vi "Launcher.vi"(8 "error in (no error)":errorcluster) -> (0 "error out":errorcluster)   [LabVIEW 2022 SP3]
doc: "This VI launches the image analyzer application."
uses:
  Controls/LauncherStates.ctl
  Test Application Controller/Test Application Controller.lvclass
  C:/Program Files/National Instruments/LabVIEW 2022/vi.lib/ActorFramework/Actor/Actor.lvclass
  <vilib>/ActorFramework/Message Enqueuer/Message Enqueuer.lvclass/Message Enqueuer.ctl
  <vilib>/ActorFramework/Message Enqueuer/Enqueue.vi
  Test Application Controller Messages/Launch UI Msg/Launch UI Msg.lvclass
  C:/Program Files/National Instruments/LabVIEW 2022/vi.lib/ActorFramework/Message/Message.lvclass
  <vilib>/ActorFramework/Message Priority Queue/Priority Enqueue.vi
  <vilib>/ActorFramework/Actor/Actor.lvclass
panel:
  out "Status":string
  out "Slide":i32(slide) scale=0.0..100.0
  # "Test Application v0.0"
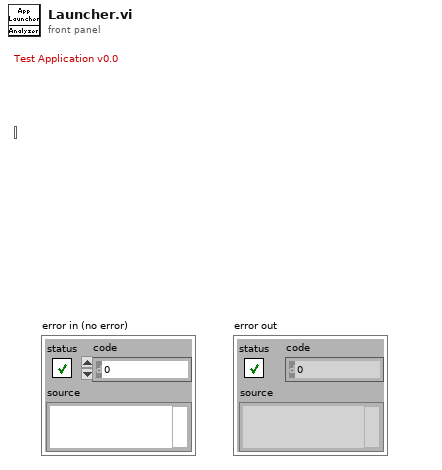
[diagram p1: front panel]
types:
  T1 = typedef "LauncherStates.ctl" = enum16{"Initialize", "Check License...", "Check Files...", "Launching Main...", "Force Stop", "Exit"}
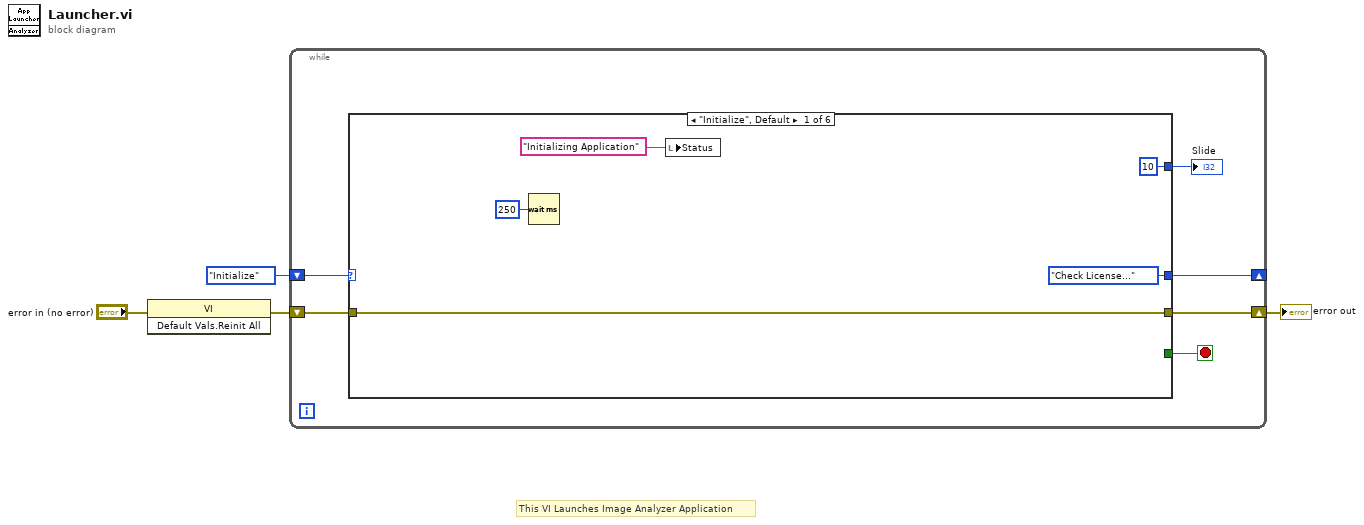
[diagram p0: block diagram]
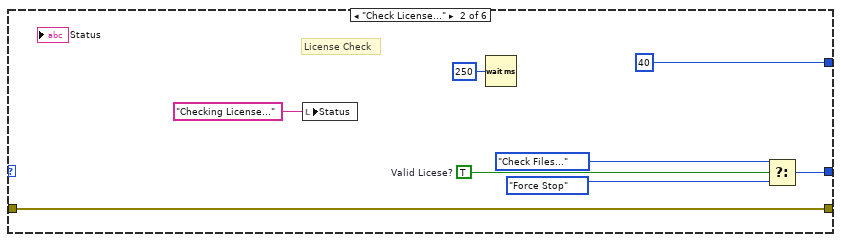
[diagram p2: hidden frame]
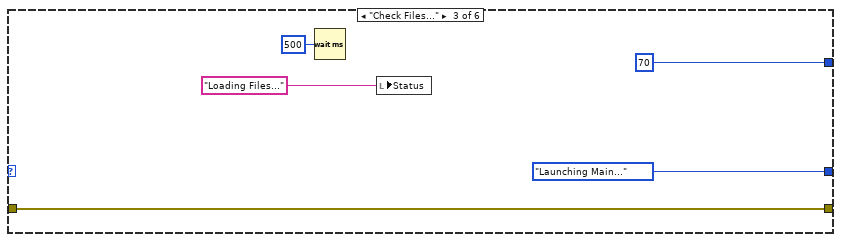
[diagram p3: hidden frame]
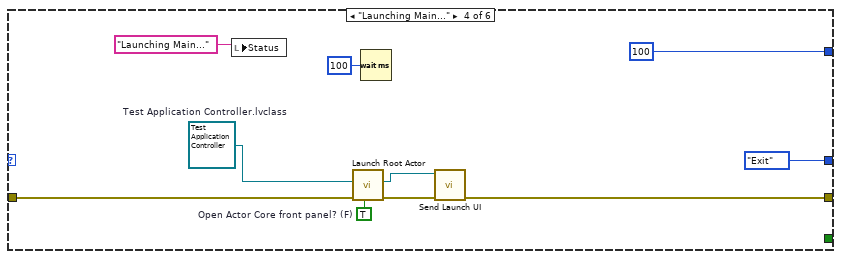
[diagram p4: hidden frame]
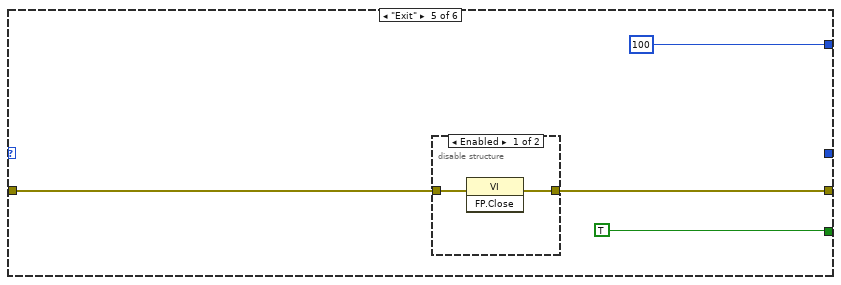
[diagram p5: hidden frame]
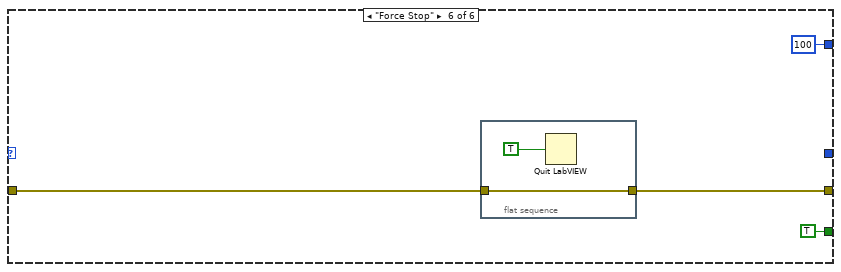
[diagram p7: hidden frame]
diagram:
  # "This VI Launches Image Analyzer Application"
  n1 = invoke class="VI" method="Default Vals.Reinit All"(error in="error in (no error)") -> (error out=w1:errorcluster)  [unwired: 2 in, 2 out]
  n2 = while {
    shift-right: [w9] -> _
    shift-left: LauncherStates."Initialize" -> [w10]
    shift-right: [w7] -> w3
    shift-left: w1 -> [w8]
    stop <- w6 stop-if-true
    n3 = case shown="\"Initialize\", Default" w10 {
      tunnel: [LauncherStates."Check License..." w21 LauncherStates."Launching Main..." LauncherStates."Exit" _ _] -> w9
      tunnel: w8 -> [w11 w18 w24 w38 w39 w45]
      tunnel: [w11 w18 w24 w30 w40 w46] -> w7
      tunnel: [_ _ _ _ TRUE TRUE] -> w6
      tunnel: [10 ("Slide") 40 ("Slide") 70 ("Slide") 100 ("Slide") 100 ("Slide") 100 ("Slide")] -> w5
      frame "Initialize", Default {
        n4 = Wait (ms)(milliseconds to wait=u32 250) -> ()  [unwired: 1 out]
        n5 = local write "Status"("Initializing Application" ("Status")) -> ()
      }
      frame "Check License..." {
        w17 = TRUE  # Valid Licese?
        # "License Check"
        n6 = local write "Status"("Checking License..." ("Status")) -> ()
        n7 = Wait (ms)(milliseconds to wait=u32 250) -> ()  [unwired: 1 out]
        n8 = Select(t=LauncherStates."Check Files...", s=w17, f=LauncherStates."Force Stop") -> (s? t:f=w21:T1)
      }
      frame "Check Files..." {
        n9 = Wait (ms)(milliseconds to wait=u32 500) -> ()  [unwired: 1 out]
        n10 = local write "Status"("Loading Files..." ("Status")) -> ()
      }
      frame "Launching Main..." {
        w32 = refnum<class "Test Application Controller.lvclass"> refnum  # Test Application Controller.lvclass
        w33 = TRUE  # Open Actor Core front panel? (F)
        n11 = local write "Status"("Launching Main..." ("Status")) -> ()
        n12 = call <vilib>:"Launch Root Actor.vi"("Open Actor Core front panel? (F)"=w33, "error in (no error)"=w38, "Actor"=w32) -> ("error out"=w31:errorcluster, "Actor's Enqueuer"=w29:refnum<class "Message Enqueuer.lvclass">)  [unwired: 7 in]
        n13 = Wait (ms)(milliseconds to wait=u32 100) -> ()  [unwired: 1 out]
        n14 = call "Send Launch UI.vi"("error in (no error)"=w31, "Message Enqueuer"=w29) -> ("error out"=w30:errorcluster)  [unwired: 8 in, 1 out]
      }
      frame "Exit" {
        n15 = disable-structure shown="Enabled" {
          disable-tunnel: [w44 _] -> w40
          disable-tunnel: w39 -> [w43 _]
          frame Enabled {
            n16 = invoke class="VI" method="FP.Close"(error in=w43) -> (error out=w44:errorcluster)  [unwired: 2 in, 2 out]
          }
          frame Disabled {
          }
        }
      }
      frame "Force Stop" {
        n17 = flat-sequence {
          tunnel: w45 -> [w49]
          tunnel: [w49] -> w46
          frame #0 {
            n18 = Quit LabVIEW(quit? (T)=TRUE) -> ()
          }
        }
      }
    }
    "Slide" <- w5
  }
  "error out" <- w3
